vi "Sensors.vi"(8 "error in (no error)":errorcluster) -> (0 "error out":errorcluster, 3 "Sensors Data":T1={"Temperature (°C)"=nan, "Barometric Pressure (mbar)"=nan, "Humidity (%)"=nan, "Temperature Cooler (K)"=nan})   [LabVIEW 2019, in "ACSVcontrol-driver.lvlib"]
doc: "Measures the environmental temperature, humidity, barom. pressure and in case of a cryocooler system the cooler temperature too."
uses:
  ACSVcontrol-driver.lvlib
  Type Definitions/Sensors Data.ctl
  Private/Type definitions/Status.ctl
  Private/Type definitions/Command.ctl
  Private/Type definitions/Instruction.ctl
  Private/Globals.vi
  <vilib>/Utility/error.llb/Error Cluster From Error Code.vi
  <vilib>/ErrorRing/Error Ring.xnode
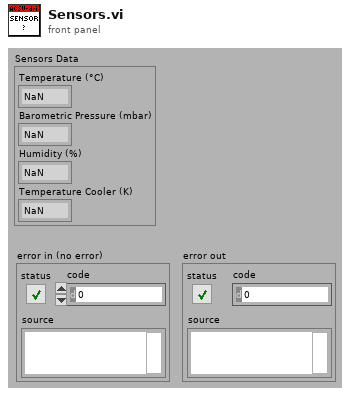
[diagram p1: front panel]
types:
  T1 = typedef "ACSVcontrol-driver.lvlib/Sensors Data.ctl" = cluster{"Temperature (°C)":dbl, "Barometric Pressure (mbar)":dbl, "Humidity (%)":dbl, "Temperature Cooler (K)":dbl}
  T2 = typedef "ACSVcontrol-driver.lvlib/Status.ctl" = enum16{"waiting", "processing", "error command", "Set_PJVS-Done", "Set_Mux-Done", "Set_Mux-Error", "Set_57XX-Done", "Set_57XX-Error", "Set_Gen-Done", "Set_Gen-Error", "Set_Synthesizer-Done", "Set_Synthesizer-Error", "Read_Nano-Done", "Read_Sampler-Done", "Read_Sampler-Error", "Read_Sensors-Done"}
  T3 = typedef "ACSVcontrol-driver.lvlib/Command.ctl" = enum16{"Set_PJVS", "Set_Mux", "Set_57XX", "Set_Gen", "Set_Synthesizer", "Read_Nulldetector", "Read_Sampler", "Read_Sensors"}
  T4 = typedef "ACSVcontrol-driver.lvlib/Instruction.ctl" = enum16{"dummy - do not use", "Send Command", "Read Result", "Ask Status"}
  T5 = typedef "ACSVcontrol-driver.lvlib/Timeouts.ctl" = cluster{"TCP Read & Write (ms)":i32, "Sensors readout":i32, "PJVS setup":i32, "Nullmeter readout":i32, "Multiplexer setup":i32, "57XX setup":i32, "Generator setup":i32, "Synthesizer setup":i32, "Sampler readout":i32}
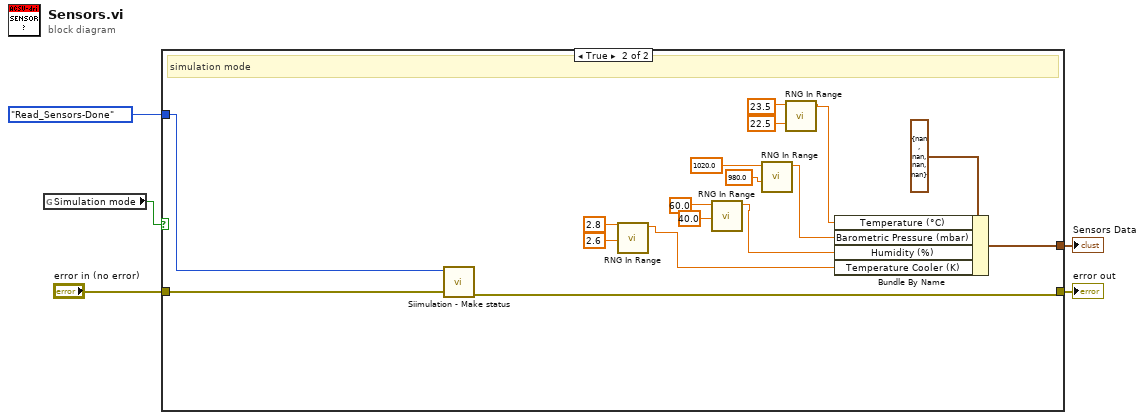
[diagram p0: block diagram]
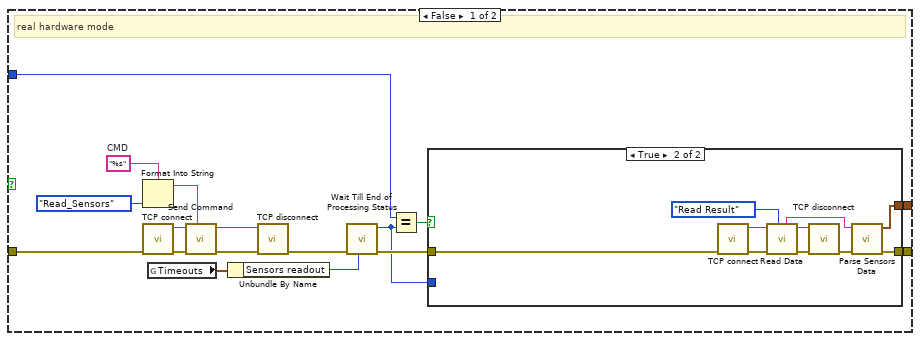
[diagram p2: hidden frame]
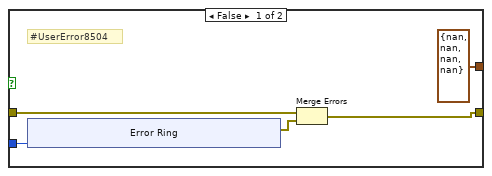
[diagram p3: hidden frame]
diagram:
  n1 = global read "Globals.vi" "Simulation mode"() -> (w2:bool)
  n2 = case shown="True" w2 {
    tunnel: "error in (no error)" -> [w20 w59]
    tunnel: [w13 w58] -> w4
    tunnel: [w10 w60] -> w3
    tunnel: Status."Read_Sensors-Done" ("x") -> [w6 w57]
    frame False {
      w22 = "%s"  # CMD
      # "real hardware mode"
      n3 = Format Into String(format string=w22, Command."Read_Sensors" ("Command")) -> (resulting string=w7:string)  [unwired: 2 in, 1 out]
      n4 = call "TCP connect.vi"("error in (no error)"=w20) -> ("error out"=w19:errorcluster, "connection ID"=w18:refnum<k5>)  [unwired: 9 in]
      n5 = global read "Globals.vi" "Timeouts"() -> (w8:T5)
      n6 = call "Send Command.vi"("Command"=w7, "error in (no error)"=w19, "connection ID"=w18) -> ("error out"=w17:errorcluster, "connection ID out"=w15:refnum<k5>)  [unwired: 7 in]
      n7 = Unbundle By Name(w8) -> ("Sensors readout"=w9:i32)
      n8 = call "TCP disconnect.vi"("error in (no error)"=w17, "connection ID"=w15) -> ("error out"=w16:errorcluster)  [unwired: 9 in]
      n9 = call "Wait Till End of Processing Status.vi"("Loop Timeout (ms) (5000)"=w9, "error in (no error)"=w16) -> ("error out"=w14:errorcluster, "Last Status"=w11:T2)  [unwired: 8 in]
      n10 = Equal?(x=w6, y=w11) -> (x = y?=w12:bool)
      n11 = case shown="True" w12 {
        tunnel: w14 -> [w27 w42]
        tunnel: [w24 w38] -> w13
        tunnel: w11 -> [w26 _]
        tunnel: [T1 {"Temperature (°C)"=nan, "Barometric Pressure (mbar)"=nan, "Humidity (%)"=nan, "Temperature Cooler (K)"=nan} ("Sensors Data") w37] -> w10
        frame False {
          # "#UserError8504"
          n12 = xnode "Error Ring"("parameter 0"=w26) -> ("error out"=w25:errorcluster)
          n13 = Merge Errors(w27, w25) -> (w24:errorcluster)
        }
        frame True {
          n14 = call "TCP connect.vi"("error in (no error)"=w42) -> ("error out"=w41:errorcluster, "connection ID"=w40:refnum<k5>)  [unwired: 9 in]
          n15 = call "Read Data.vi"("Instruction"=Instruction."Read Result", "error in (no error)"=w41, "connection ID"=w40) -> ("error out"=w44:errorcluster, "connection ID out"=w43:refnum<k5>, "Data"=w35:string)  [unwired: 6 in]
          n16 = call "TCP disconnect.vi"("error in (no error)"=w44, "connection ID"=w43) -> ("error out"=w39:errorcluster)  [unwired: 9 in]
          n17 = call "Parse Sensors Data.vi"("error in"=w39, "Data"=w35) -> ("error out"=w38:errorcluster, "Sensors Data"=w37:T1)  [unwired: 8 in]
        }
      }
    }
    frame True {
      # "simulation mode"
      n18 = call "Siimulation - Make status.vi"("error in (no error)"=w59, "Status"=w57) -> ("error out"=w58:errorcluster)  [unwired: 8 in, 1 out]
      n19 = call "RNG In Range.vi"("llimit 2 (1)"=2.6 ("lower bound (0)"), "limit 1 (0)"=2.8 ("upper bound (100)")) -> ("number"=w45:dbl)  [unwired: 9 in]
      n20 = call "RNG In Range.vi"("llimit 2 (1)"=40.0 ("lower bound (0)"), "limit 1 (0)"=60.0 ("upper bound (100)")) -> ("number"=w49:dbl)  [unwired: 9 in]
      n21 = call "RNG In Range.vi"("llimit 2 (1)"=980.0 ("lower bound (0)"), "limit 1 (0)"=1020.0 ("upper bound (100)")) -> ("number"=w53:dbl)  [unwired: 9 in]
      n22 = call "RNG In Range.vi"("llimit 2 (1)"=22.5 ("lower bound (0)"), "limit 1 (0)"=23.5 ("upper bound (100)")) -> ("number"=w54:dbl)  [unwired: 9 in]
      n23 = Bundle By Name(cluster=T1 {"Temperature (°C)"=nan, "Barometric Pressure (mbar)"=nan, "Humidity (%)"=nan, "Temperature Cooler (K)"=nan} ("Sensors Data"), "Temperature (°C)"=w54, "Barometric Pressure (mbar)"=w53, "Humidity (%)"=w49, "Temperature Cooler (K)"=w45) -> (w60:T1)
    }
  }
  "error out" <- w4
  "Sensors Data" <- w3
